vi "ArmControlTemp.vi"(8 "error in":errorcluster) -> ()   [LabVIEW 2014]
uses:
  <vilib>/Rock Robotics/WPI/Joystick/WPI_JoystickGetSetRefNum.vi
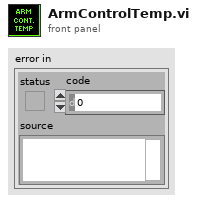
[diagram p1: front panel]
types:
  T1 = typedef "WPI_JoystickDevRef.ctl" = cluster{"Device":T2}
  T2 = typedef "WPI_JoystickDeviceEnum.ctl" = enum16{"USB 0", "USB 1", "USB 2", "USB 3", "USB 4", "USB 5"}
  T3 = typedef "WPI_MotorControlDeviceRef.ctl" = cluster{"DeviceStatus":errorcluster, "Type":T4, "PWM":cluster{"Controller":T5, "PWM Channel":T6, "DeadBand":T7}, "CAN":cluster{"Device Number":u8, "Control Mode":T8, "Semaphore":T9, "Max Vout":dbl, "TalonSRX Control Mode":T10}, "Invert":bool, "TransformRef":T11, "InvTransformRef":T11}
  T4 = typedef "WPI_MotorControlType.ctl" = enum16{"PWM", "CAN", "CANTalonSRX"}
  T5 = typedef "FPGA_TypedefDigitalModule.ctl" = enum16{"Controller 1"}
  T6 = typedef "FPGA_DIOPWMChannel.ctl" = enum8{"PWM 0", "PWM 1", "PWM 2", "PWM 3", "PWM 4", "PWM 5", "PWM 6", "PWM 7", "PWM 8", "PWM 9", "PWM MXP 0", "PWM MXP 1", "PWM MXP 2", "PWM MXP 3", "PWM MXP 4", "PWM MXP 5", "PWM MXP 6", "PWM MXP 7", "PWM MXP 8", "PWM MXP 9", "Invalid"}
  T7 = typedef "WPI_PWMDeadband.ctl" = cluster{"Name":string, "maxPositivePwm":i32, "minPositivePwm":i32, "centerPwm":i32, "maxNegativePwm":i32, "minNegativePwm":i32, "angularRange":u16}
  T8 = typedef "WPI_CANJaguar_ControlMode.ctl" = enum8{"Percent VBus", "Current", "Speed", "Position", "Voltage"}
  T9 = typedef "Semaphore RefNum" = refnum<k1>
  T10 = typedef "WPI_CANTalonSRX_APIControlMode.ctl" = enum8{"Percent VBus", "Speed", "Position", "Slave", "Unchanged / Invalid"}
  T11 = typedef "WPI_PWMTransform_ConPane.ctl" = refnum<vi>
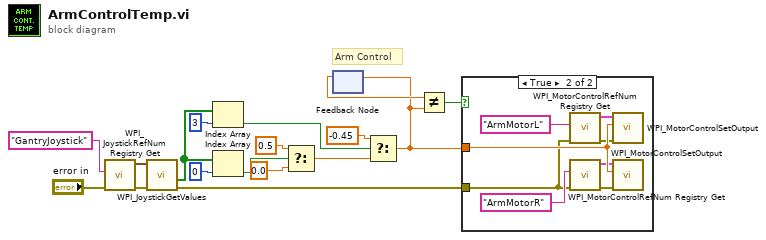
[diagram p0: block diagram]
diagram:
  # "Arm Control"
  n1 = call <vilib>:"WPI_JoystickRefNum Registry Get.vi"("error in (no error)"="error in", "refnum name"="GantryJoystick") -> ("error out"=w17:errorcluster, "JoystickDevRef"=w16:T1)  [unwired: 8 in]
  n2 = call <vilib>:"WPI_JoystickGetValues.vi"("error in (no error)"=w17, "JoystickDevRef"=w16) -> ("error out"=w1:errorcluster, "Buttons"=w6:bool[])  [unwired: 5 in, 3 out]
  n3 = Index Array(array=w6, index=3) -> (element=w5:bool)
  n4 = Index Array(array=w6, index=0) -> (element=w12:bool)
  n5 = Select(t=0.5, s=w12, f=0.0) -> (s? t:f=w11:dbl)
  n6 = feedback #1() -> (w3:dbl)  [unwired: 1 in]
  n7 = Select(t=-0.45, s=w5, f=w11) -> (s? t:f=w2:dbl)
  n8 = feedback-in #1(w2) -> ()
  n9 = Not Equal?(x=w3, y=w2) -> (x != y?=w4:bool)
  n10 = case shown="True" w4 {
    tunnel: w2 -> [_ w25]
    tunnel: w1 -> [_ w18]
    frame False {
    }
    frame True {
      n11 = call <vilib>:"WPI_MotorControlRefNum Registry Get.vi"("error in (no error)"=w18, "refnum name"="ArmMotorL") -> ("error out"=w21:errorcluster, "MotorControlDevRef"=w22:T3)  [unwired: 8 in]
      n12 = call <vilib>:"WPI_MotorControlRefNum Registry Get.vi"("error in (no error)"=w18, "refnum name"="ArmMotorR") -> ("error out"=w19:errorcluster, "MotorControlDevRef"=w20:T3)  [unwired: 8 in]
      n13 = call <vilib>:"WPI_MotorControlSetOutput.vi"("error in (no error)"=w21, "Output"=w25, "MotorControlDevRef"=w22) -> ()  [unwired: 6 in, 3 out]
      n14 = call <vilib>:"WPI_MotorControlSetOutput.vi"("error in (no error)"=w19, "Output"=w25, "MotorControlDevRef"=w20) -> ()  [unwired: 6 in, 3 out]
    }
  }
